vi "_SBR_mes_PM.vi"(6 "SBR_Set":T3={"file_name"="", "HOT/COLD AUTO"=TRUE, "MPI SSB Set"=TRUE, "AUTO時待ち時間（S）"=1.0, "P/V         V/P"=FALSE, "save"=TRUE, "start(GHz)"=4.0, "stop(GHz) "=12.0, "Step(GHz) "=0.1, "P.M.aveg"=10, "PM        SP"=FALSE, "SP_set"={"start(GHz)"=3.5, "stop(GHz) "=12.5, "BW(MHz)"=8.0, "VBW(Hz)"=30.0, "ref(dBm)"=-45.0, "log(dB)"=1.0, "AVEG"=1, "AVEG ON/OFF"=FALSE, "Auto Align ON/OFF"=FALSE, "GPIB"="18", "point"=801}}, 7 "Control":T2={"GPIB_ATT"="28", "6501Dev#"=1, "GPIB_SP"="18", "GPIB_PM"="13", "GPIB_DSA"="11", "GPIB_DMM (TPD)"="23", "MPICOM"="COM5", "mortor設定"=[{"Axis"=0, "ID"=0, "HIspeed"=200.0, "LOspeed"=100.0, "ACCEL(ms)"=100.0, "Sratio"=50.0, "フリーラン\n"=FALSE, "文字列"="DSB HOT/COLD"}, {"Axis"=1, "ID"=0, "HIspeed"=4.0, "LOspeed"=4.0, "ACCEL(ms)"=100.0, "Sratio"=50.0, "フリーラン\n"=TRUE, "文字列"="SubMM Att"}, {"Axis"=0, "ID"=0, "HIspeed"=200.0, "LOspeed"=100.0, "ACCEL(ms)"=100.0, "Sratio"=50.0, "フリーラン\n"=FALSE, "文字列"="MPI Port1"}, {"Axis"=1, "ID"=0, "HIspeed"=200.0, "LOspeed"=100.0, "ACCEL(ms)"=100.0, "Sratio"=50.0, "フリーラン\n"=FALSE, "文字列"="MPI Port2"}], "DATAパス"=path "C:/Documents and Settings/?澤佳?/デスクトップ/data/プロトカ?トリッジ/100811_protC4-5/100814_WCA_P0", "DBパス "=path "Z:/band10/Labview_ALMA/MIX95/test", "comment"="NOLO", "ColdCarts"="003601", "Th"=295.0, "Tc"=77.0, "Set_SIS_volt"=2.096774193548387, "Offset"=0.0, "control"=0, "FreqLO"=796.0, "Set_Mag_Cur"=800.0, "MPI offset(mm)"=22.99, "HOT/COLD"=0} {"HOT/COLD" items=["DSB", "SBR", "GainComp"]; "control" items=["CLOSE LOOP", "OPEN LOOP", "Not Control"]}) -> ()   [LabVIEW 2017]
uses:
  <vilib>/express/express arith-compare/Formula/XNode/ExpressFormulaBlockNode.xnode
panel:
  out "XYグラフ 5":cluster{"データ配列":dbl[], "データ配列":dbl[]}[](graph)
  out "XYグラフ 3":cluster{"データ配列":dbl[], "データ配列":dbl[]}[](graph)=[{"データ配列"=[846.0, 845.9, 845.8, 845.7, 845.6, 845.5, 845.4, 845.3, 845.2, 845.1, 845.0, 844.9, 844.8, 844.7, 844.6, 844.5, 844.4, 844.3, 844.2, 844.1, 844.0, 843.9, 843.8, 843.7, 843.6, 843.5, 843.4, 843.3, 843.2, 843.1, 843.0, 842.9, 842.8, 842.7, 842.6, 842.5, 842.4, 842.3, 842.2, 842.1, 842.0, 841.9, 841.8, 841.7, 841.6, 841.5, 841.4, 841.3, 841.2, 841.1, 841.0, 840.9, 840.8, 840.7, 840.6, 840.5, 840.4, 840.3, 840.2, 840.1, 840.0, 839.9, 839.8, 839.7, 839.6, 839.5, 839.4, 839.3, 839.2, 839.1, 839.0, 838.9, 838.8, 838.7, 838.6, 838.5, 838.4, 838.3, 838.2, 838.1, 838.0], "データ配列"=[548.6440300868269, 532.3446978159301, 548.2566145023541, 544.9061292459833, 538.3138371670094, 526.7499707435629, 519.9997703838006, 527.593359910926, 538.6649629641214, 528.8783476971857, 531.9759636549385, 528.4548463210765, 513.5100557424433, 516.344277513952, 524.5874165109195, 514.3547194297134, 503.7653656940615, 515.5843212692465, 511.0783598537313, 507.55375171659057, 505.8555142030906, 497.52972774878066, 501.23367501224743, 498.1244938121795, 489.8630053526426, 493.1999495623687, 486.236254971209, 488.3096964717638, 482.9518498217425, 485.03073723710247, 486.70267213607735, 480.58951323335924, 482.1108023321396, 481.7962553542322, 480.2342668763604, 480.1246358814105, 478.34749024616036, 479.50312619911205, 480.8342642556151, 480.11632993657906, 480.09010262034064, 481.33419008499317, 479.94632437429556, 479.2444411258671, 475.56007043143904, 479.92516925660385, 474.2701582066877, 475.40266728367556, 479.1159951944159, 479.7010196459051, 475.52458759109373, 472.89567054194913, 473.80662563539966, 472.1704784340717, 468.6585989006322, 468.80409014491283, 479.386903232559, 475.6610934283412, 469.07237974406974, 469.8923820760799, 485.7474282618513, 474.9909858241797, 477.7451890508568, 471.7345659278333, 466.80799840032967, 476.31289425549187, 474.0855612238338, 468.51643935953587, 465.4725917144067, 464.39387004779314, 455.68701805229597, 487.4824379927386, 486.6396397044617, 482.6491011961885, 476.185717770886, 473.69367551401047, 469.2462719814977, 490.9878049262109, 488.417091028331, 483.2977332637604, 478.73867571328907]}, {"データ配列"=[854.0, 854.1, 854.2, 854.3, 854.4, 854.5, 854.6, 854.7, 854.8, 854.9, 855.0, 855.1, 855.2, 855.3, 855.4, 855.5, 855.6, 855.7, 855.8, 855.9, 856.0, 856.1, 856.2, 856.3, 856.4, 856.5, 856.6, 856.7, 856.8, 856.9, 857.0, 857.1, 857.2, 857.3, 857.4, 857.5, 857.6, 857.7, 857.8, 857.9, 858.0, 858.1, 858.2, 858.3, 858.4, 858.5, 858.6, 858.7, 858.8, 858.9, 859.0, 859.1, 859.2, 859.3, 859.4, 859.5, 859.6, 859.7, 859.8, 859.9, 860.0, 860.1, 860.2, 860.3, 860.4, 860.5, 860.6, 860.7, 860.8, 860.9, 861.0, 861.1, 861.2, 861.3, 861.4, 861.5, 861.6, 861.7, 861.8, 861.9, 862.0], "データ配列"=[428.63466788231324, 435.4935786985518, 424.9429241146229, 425.381002919813, 433.20647623071613, 438.7104620965752, 443.67374232684676, 442.41046901070797, 430.10206610123777, 440.4868132571015, 435.759630172149, 438.12370344225775, 449.17411817434277, 446.7229210528855, 440.15843962648995, 446.8897154052984, 455.8583559850793, 448.5867165832221, 448.7198763169121, 459.213527054518, 453.52958129721236, 461.1908621778645, 460.27576536783874, 460.2582724546055, 466.0864670209972, 465.7857212585232, 472.4310313017354, 469.17709649506514, 472.78362850317023, 474.8300149659003, 470.5899912757829, 476.0942267925349, 475.8579793140339, 477.7303156869513, 475.74400495243003, 477.79647352046953, 480.42504158528186, 480.43932637294694, 476.7091000205245, 476.62383716173747, 478.55303619667967, 475.9076566852461, 479.478478145908, 479.03123367121594, 482.39234918165187, 479.54022383471187, 482.5907823874182, 481.7505278760315, 473.16388160930836, 478.15362306779105, 480.4224566467349, 486.5333822347131, 481.63681143700416, 483.9492838089557, 486.8070352464491, 488.59582820525645, 476.5343014109415, 481.9312913888416, 483.0061248872076, 487.93423410039685, 474.129463031071, 479.9925386625467, 481.15577320464706, 486.42199876382404, 486.19935785269905, 480.1111428291795, 482.85166491000814, 488.0712289584561, 488.79712182957707, 494.7195539445724, 498.2972613667672, 469.3853698503216, 471.69756792095194, 474.9496602642304, 474.9261101258189, 481.58901751620425, 485.18240521858206, 464.0725253238966, 468.63537032154585, 470.95286464714934, 473.82427991781964]}]
  out "XYグラフ 2":cluster{"データ配列":dbl[], "データ配列":dbl[]}[](graph)=[{"データ配列"=[4.0, 4.1, 4.2, 4.3, 4.4, 4.5, 4.6, 4.7, 4.8, 4.9, 5.0, 5.1, 5.2, 5.3, 5.4, 5.5, 5.6, 5.7, 5.8, 5.9, 6.0, 6.1, 6.2, 6.3, 6.4, 6.5, 6.6, 6.7, 6.8, 6.9, 7.0, 7.1, 7.2, 7.3, 7.4, 7.5, 7.6, 7.7, 7.8, 7.9, 8.0, 8.1, 8.2, 8.3, 8.4, 8.5, 8.6, 8.7, 8.8, 8.9, 9.0, 9.1, 9.2, 9.3, 9.4, 9.5, 9.6, 9.7, 9.8, 9.9, 10.0, 10.1, 10.2, 10.3, 10.4, 10.5, 10.6, 10.7, 10.8, 10.9, 11.0, 11.1, 11.2, 11.3, 11.4, 11.5, 11.6, 11.7, 11.8, 11.9, 12.0], "データ配列"=[0.9249046199806905, 0.7517460823312963, 0.9540395840198505, 0.9269162846964503, 0.8135071464293695, 0.6845118078872291, 0.5940848741555105, 0.6595267429496003, 0.8424905890766325, 0.6848614491447951, 0.7468632569240828, 0.7017022540247116, 0.5009781568393058, 0.5420517670471693, 0.6567512705093524, 0.5260819433781404, 0.3738892851233047, 0.5210577608576411, 0.4868080144723247, 0.3748668646829679, 0.40851305214688144, 0.2837618549546105, 0.31906128888492447, 0.29578752754072546, 0.186091340659989, 0.21398760146405285, 0.10777417863579805, 0.149529503683046, 0.07958880444948759, 0.07954748815261764, 0.1259459192415544, 0.03515471930494699, 0.048843010718681204, 0.03171586659857754, 0.03513774392157607, 0.01818671370440185, -0.01621661399776954, -0.007299958166486085, 0.03223525679436591, 0.02731107388958061, 0.01199917327442536, 0.042416189630546657, 0.003649695010670608, 0.0016649617408312201, -0.05337023868420484, 0.003002871580193121, -0.06506068611910158, -0.049621795287776015, 0.046733111271247955, 0.012088382838128539, -0.038328518852154166, -0.10639347213811458, -0.061303944619701796, -0.09216414898512537, -0.14209487210153343, -0.15469411614691805, 0.022323601941448917, -0.04899532047290484, -0.10942566444854036, -0.14096019154058603, 0.0905989021163112, -0.0391739187880516, -0.026618766005445365, -0.11471481804298753, -0.1521656000206294, -0.02971053894241202, -0.06853941673839113, -0.15295352656935207, -0.18282933440970475, -0.23669712055460096, -0.33420193764281625, 0.14151372779511212, 0.11668493408571631, 0.06016340251879209, 0.00990019059975937, -0.06182303914612333, -0.12488763229092192, 0.2108352941071432, 0.1546641658899227, 0.09675663767559298, 0.0385754646352136]}, {"データ配列"=[4.0, 4.1, 4.2, 4.3, 4.4, 4.5, 4.6, 4.7, 4.8, 4.9, 5.0, 5.1, 5.2, 5.3, 5.4, 5.5, 5.6, 5.7, 5.8, 5.9, 6.0, 6.1, 6.2, 6.3, 6.4, 6.5, 6.6, 6.7, 6.8, 6.9, 7.0, 7.1, 7.2, 7.3, 7.4, 7.5, 7.6, 7.7, 7.8, 7.9, 8.0, 8.1, 8.2, 8.3, 8.4, 8.5, 8.6, 8.7, 8.8, 8.9, 9.0, 9.1, 9.2, 9.3, 9.4, 9.5, 9.6, 9.7, 9.8, 9.9, 10.0, 10.1, 10.2, 10.3, 10.4, 10.5, 10.6, 10.7, 10.8, 10.9, 11.0, 11.1, 11.2, 11.3, 11.4, 11.5, 11.6, 11.7, 11.8, 11.9, 12.0], "データ配列"=[0.8608442548458806, 0.7044947061255087, 0.942586230446133, 0.8493423462533632, 0.7498852904990045, 0.6081560581526015, 0.5430236262647461, 0.6112878364871215, 0.7766440219127979, 0.6149782219119803, 0.6572667110064123, 0.6314153665922547, 0.42698388986216995, 0.42556280195907853, 0.6250719853321322, 0.46430207183002675, 0.33449694284816134, 0.3882474607513784, 0.41506556549956136, 0.3095955000245737, 0.3439051059443347, 0.18240325622893133, 0.28216500097201935, 0.21140353248088684, 0.09413496569057882, 0.17821059451244267, 0.02989001559470223, 0.08828842570711844, 0.050866182648811285, 0.05573387700815249, 0.0663662835217892, 0.0060675597842494156, 0.025335116139840193, -0.04466065840811484, -0.0009333943257959284, -0.05014719752768275, -0.03863850457661142, -0.05952305731929579, -0.037721361400900405, -0.057166062404831075, -0.02916814808995304, -0.012193201434749976, -0.05312032998266237, -0.03611908754398227, -0.1487916724233145, -0.0936345982389959, -0.11305505580370279, -0.1339112513602761, -0.06524335069777229, -0.05628499636478335, -0.11671426437024365, -0.12007755334931655, -0.07430213142730542, -0.1433316372459072, -0.19742493600277894, -0.24364724201221805, -0.08095792610453033, -0.11881261902412663, -0.18295836886949077, -0.1796637370590902, -0.0021771227974171498, -0.026775088377075353, -0.0733922953710137, -0.21148011251519863, -0.21732805814513603, -0.10245993628641197, -0.15420496911591877, -0.19693792604968408, -0.25066612288482537, -0.32217008482607234, -0.39040508822987946, 0.10341354358296367, 0.0815119128548301, -0.0023439054432579094, -0.09006479558012595, -0.1407232856746613, -0.1823207569229413, 0.17679562449456773, 0.08239435268162094, 0.017011997383429706, -0.016509469169492315]}]
  out "XYグラフ 4":cluster{"データ配列":dbl[], "データ配列":dbl[]}[](graph)=[{"データ配列"=[4.0, 4.1, 4.2, 4.3, 4.4, 4.5, 4.6, 4.7, 4.8, 4.9, 5.0, 5.1, 5.2, 5.3, 5.4, 5.5, 5.6, 5.7, 5.8, 5.9, 6.0, 6.1, 6.2, 6.300000000000001, 6.4, 6.5, 6.6, 6.7, 6.800000000000001, 6.9, 7.0, 7.1, 7.2, 7.300000000000001, 7.4, 7.5, 7.6, 7.7, 7.800000000000001, 7.9, 8.0, 8.100000000000001, 8.2, 8.3, 8.4, 8.5, 8.600000000000001, 8.7, 8.8, 8.9, 9.0, 9.100000000000001, 9.2, 9.3, 9.4, 9.5, 9.600000000000001, 9.7, 9.8, 9.9, 10.0, 10.100000000000001, 10.2, 10.3, 10.4, 10.5, 10.600000000000001, 10.7, 10.8, 10.9, 11.0, 11.100000000000001, 11.2, 11.3, 11.4, 11.5, 11.600000000000001, 11.7, 11.8, 11.9, 12.0], "データ配列"=[-12.8167177, -12.8141441, -12.8129357, -12.8127695, -12.8146098, -12.8149315, -12.8129768, -12.8171079, -12.8151768, -12.8168376, -12.8133399, -12.8138484, -12.8165291, -12.82274, -12.8215599, -12.8278529, -12.8327051, -12.84042, -12.8387483, -12.8518869, -12.8490208, -12.8535159, -12.8552697, -12.8598767, -12.8577317, -12.8589288, -12.8659834, -12.8643617, -12.866542, -12.8707753, -12.8715886, -12.8749385, -12.8803226, -12.8889543, -12.888898, -12.8977837, -12.8968323, -12.9040674, -12.9085005, -12.9114525, -12.9163973, -12.910995, -12.9094349, -12.9092876, -12.9091013, -12.9068352, -12.9020569, -12.9040377, -12.8989597, -12.899771, -12.8980538, -12.8942882, -12.8828067, -12.8807576, -12.8755902, -12.8728258, -12.8664256, -12.8622031, -12.85197, -12.8488996, -12.8492387, -12.838981799999999, -12.8414434, -12.8447165, -12.8376775, -12.840512, -12.8396292, -12.8369379, -12.8346457, -12.8405822, -12.8328279, -12.8329255, -12.8308305, -12.8282862, -12.8235474, -12.821384, -12.8175541, -12.8162696, -12.8153706, -12.8112541, -12.8080699]}, {"データ配列"=[4.0, 4.1, 4.2, 4.3, 4.4, 4.5, 4.6, 4.7, 4.8, 4.9, 5.0, 5.1, 5.2, 5.3, 5.4, 5.5, 5.6, 5.7, 5.8, 5.9, 6.0, 6.1, 6.2, 6.300000000000001, 6.4, 6.5, 6.6, 6.7, 6.800000000000001, 6.9, 7.0, 7.1, 7.2, 7.300000000000001, 7.4, 7.5, 7.6, 7.7, 7.800000000000001, 7.9, 8.0, 8.100000000000001, 8.2, 8.3, 8.4, 8.5, 8.600000000000001, 8.7, 8.8, 8.9, 9.0, 9.100000000000001, 9.2, 9.3, 9.4, 9.5, 9.600000000000001, 9.7, 9.8, 9.9, 10.0, 10.100000000000001, 10.2, 10.3, 10.4, 10.5, 10.600000000000001, 10.7, 10.8, 10.9, 11.0, 11.100000000000001, 11.2, 11.3, 11.4, 11.5, 11.600000000000001, 11.7, 11.8, 11.9, 12.0], "データ配列"=[-13.7683758, -13.7922764, -13.7633268, -13.7678909, -13.7828507, -13.8025731, -13.8131615, -13.8053932, -13.7812508, -13.8023359, -13.7920552, -13.7989576, -13.8295585, -13.8300327, -13.8131129, -13.8384301, -13.8642177, -13.8495674, -13.8552811, -13.8790433, -13.8758927, -13.8977266, -13.892538, -13.9026757, -13.916412, -13.9124923, -13.9338423, -13.9277004, -13.9399338, -13.9424098, -13.9378287, -13.9546529, -13.9572289, -13.9670513, -13.969147, -13.9785946, -13.9824585, -13.9877933, -13.9872335, -13.9922533, -13.9981255, -13.9884289, -13.9918875, -13.992756, -13.9997441, -13.98919, -13.9960103, -13.9950765, -13.9790547, -13.9820422, -13.9886454, -13.9916958, -13.9764347, -13.9790154, -13.9814203, -13.9784988, -13.9476282, -13.9532534, -13.9552977, -13.9526629, -13.9176991, -13.9298424, -13.9285866, -13.9449108, -13.9459258, -13.927964, -13.9333817, -13.9436702, -13.9472559, -13.9575221, -13.9665371, -13.8965286, -13.8978142, -13.9040012, -13.9102852, -13.9152088, -13.9199899, -13.8711522, -13.8776705, -13.8837972, -13.8899317]}, {"データ配列"=[4.0, 4.1, 4.2, 4.3, 4.4, 4.5, 4.6, 4.7, 4.8, 4.9, 5.0, 5.1, 5.2, 5.3, 5.4, 5.5, 5.6, 5.7, 5.8, 5.9, 6.0, 6.1, 6.2, 6.300000000000001, 6.4, 6.5, 6.6, 6.7, 6.800000000000001, 6.9, 7.0, 7.1, 7.2, 7.300000000000001, 7.4, 7.5, 7.6, 7.7, 7.800000000000001, 7.9, 8.0, 8.100000000000001, 8.2, 8.3, 8.4, 8.5, 8.600000000000001, 8.7, 8.8, 8.9, 9.0, 9.100000000000001, 9.2, 9.3, 9.4, 9.5, 9.600000000000001, 9.7, 9.8, 9.9, 10.0, 10.100000000000001, 10.2, 10.3, 10.4, 10.5, 10.600000000000001, 10.7, 10.8, 10.9, 11.0, 11.100000000000001, 11.2, 11.3, 11.4, 11.5, 11.600000000000001, 11.7, 11.8, 11.9, 12.0], "データ配列"=[-15.3373199, -15.3434384, -15.3418441, -15.3453406, -15.3400846, -15.3458539, -15.3440331, -15.3394241, -15.3465619, -15.3410986, -15.3426298, -15.3434557, -15.346694, -15.3533297, -15.3527599, -15.3611371, -15.3653082, -15.3685527, -15.3735164, -15.3722621, -15.3827205, -15.3861695, -15.3836614, -15.3932886, -15.3939993, -15.3902446, -15.3969746, -15.3976586, -15.402461, -15.3995764, -15.4050633, -15.4090926, -15.4122846, -15.4181912, -15.4242723, -15.4297683, -15.4273514, -15.4325704, -15.4411621, -15.4454937, -15.4471412, -15.4441903, -15.4388196, -15.4406587, -15.4410973, -15.4361552, -15.4359821, -15.4374129, -15.4407749, -15.4318682, -15.4334771, -15.4239621, -15.4191743, -15.4160723, -15.4123312, -15.4063207, -15.4018825, -15.3948126, -15.3943757, -15.3815451, -15.378063, -15.3760794, -15.371747, -15.3766317, -15.3787598, -15.3750977, -15.3734286, -15.3718175, -15.3738011, -15.3719326, -15.3744687, -15.3672418, -15.3624387, -15.360924, -15.3673373, -15.3580207, -15.3559741, -15.3543332, -15.3494625, -15.3498174, -15.3493734]}, {"データ配列"=[4.0, 4.1, 4.2, 4.3, 4.4, 4.5, 4.6, 4.7, 4.8, 4.9, 5.0, 5.1, 5.2, 5.3, 5.4, 5.5, 5.6, 5.7, 5.8, 5.9, 6.0, 6.1, 6.2, 6.300000000000001, 6.4, 6.5, 6.6, 6.7, 6.800000000000001, 6.9, 7.0, 7.1, 7.2, 7.300000000000001, 7.4, 7.5, 7.6, 7.7, 7.800000000000001, 7.9, 8.0, 8.100000000000001, 8.2, 8.3, 8.4, 8.5, 8.600000000000001, 8.7, 8.8, 8.9, 9.0, 9.100000000000001, 9.2, 9.3, 9.4, 9.5, 9.600000000000001, 9.7, 9.8, 9.9, 10.0, 10.100000000000001, 10.2, 10.3, 10.4, 10.5, 10.600000000000001, 10.7, 10.8, 10.9, 11.0, 11.100000000000001, 11.2, 11.3, 11.4, 11.5, 11.600000000000001, 11.7, 11.8, 11.9, 12.0], "データ配列"=[-14.0196387, -13.9979183, -14.0309121, -14.018873, -14.0036354, -13.9857556, -13.9744838, -13.9850344, -14.0105081, -13.9859785, -13.9904136, -13.9872409, -13.9607929, -13.9671506, -13.9949353, -13.9786552, -13.9646952, -13.9787962, -13.9830638, -13.9758055, -13.9829474, -13.9637367, -13.9786938, -13.9745032, -13.9572288, -13.9680508, -13.9544577, -13.9613969, -13.9599726, -13.9615707, -13.9660668, -13.960714, -13.9681177, -13.9661289, -13.9740149, -13.975349, -13.9750328, -13.9785234, -13.9884027, -13.9882046, -13.9960013, -13.9947386, -13.9851271, -13.9880813, -13.9730589, -13.9769712, -13.9707784, -13.9701434, -13.9780513, -13.9759535, -13.96688, -13.9613857, -13.9585451, -13.9457407, -13.9334979, -13.9238702, -13.9411322, -13.9297898, -13.9138048, -13.9083049, -13.933475, -13.9215995, -13.9145318, -13.8989468, -13.8948861, -13.9126915, -13.9031456, -13.8942396, -13.8858065, -13.8794991, -13.8666928, -13.9337306, -13.926695, -13.9122424, -13.8990967, -13.8877931, -13.8797191, -13.9291645, -13.9124584, -13.900162, -13.8931044]}, {"データ配列"=[4.0, 4.1, 4.2, 4.3, 4.4, 4.5, 4.6, 4.7, 4.8, 4.9, 5.0, 5.1, 5.2, 5.3, 5.4, 5.5, 5.6, 5.7, 5.8, 5.9, 6.0, 6.1, 6.2, 6.300000000000001, 6.4, 6.5, 6.6, 6.7, 6.800000000000001, 6.9, 7.0, 7.1, 7.2, 7.300000000000001, 7.4, 7.5, 7.6, 7.7, 7.800000000000001, 7.9, 8.0, 8.100000000000001, 8.2, 8.3, 8.4, 8.5, 8.600000000000001, 8.7, 8.8, 8.9, 9.0, 9.100000000000001, 9.2, 9.3, 9.4, 9.5, 9.600000000000001, 9.7, 9.8, 9.9, 10.0, 10.100000000000001, 10.2, 10.3, 10.4, 10.5, 10.600000000000001, 10.7, 10.8, 10.9, 11.0, 11.100000000000001, 11.2, 11.3, 11.4, 11.5, 11.600000000000001, 11.7, 11.8, 11.9, 12.0], "データ配列"=[-15.3381941, -15.344199, -15.3447699, -15.3425074, -15.3371397, -15.3411604, -15.3414315, -15.3458022, -15.3417021, -15.3392578, -15.3397076, -15.3444271, -15.3474302, -15.3513504, -15.3547842, -15.3633021, -15.3614004, -15.3666426, -15.3702935, -15.3730672, -15.379985, -15.3834281, -15.3866312, -15.3912841, -15.3891415, -15.3940469, -15.3981261, -15.3947827, -15.3998376, -15.4000821, -15.408751, -15.4094613, -15.4119679, -15.417087, -15.4276622, -15.4229367, -15.429126, -15.4411081, -15.4378729, -15.4476114, -15.4489349, -15.4440339, -15.44137, -15.4421306, -15.434502, -15.4333984, -15.4405416, -15.4352283, -15.4339626, -15.4288343, -15.4309286, -15.422514, -15.4216582, -15.4149915, -15.4117796, -15.3984203, -15.4001348, -15.3945141, -15.3895448, -15.3827213, -15.3762016, -15.3734612, -15.3759497, -15.3702058, -15.3743928, -15.3765457, -15.3732681, -15.3712204, -15.3747897, -15.3710142, -15.3719226, -15.3681146, -15.3646886, -15.3646273, -15.3572943, -15.3592383, -15.3537235, -15.354729, -15.3478549, -15.3463945, -15.3471664]}]
  out "文字列":string="19.85991\r\n"
  in  "Tin":T1(ring)
  in  "OKボタン":bool=TRUE
  in  "タブ制御器":enum32{"ページ 5", "ページ 2", "ページ 4"}(tab)
  out "MPI SBR(dB)":dbl=19.65107286127357
  out "MU（mag）":dbl=0.6324558993924078
  out "ML（mag）":dbl=0.006853666405205144
  out "MPIPOS（mm）":dbl=19.85991633178654
  out "1Dデータ":dbl[](array[numeric])=[12.0, -12.8080699, -13.8899317, -15.3493734, -13.8931044, -15.3471664, 19.85991633178654, 0.0]
  out "SBRAクラスタ":T4={"データ配列"=array801x17[13617 elements], "Points"=801, "Th"=297.0, "Tc"=77.0, "LO(GHz)"=0.0, "Offset(mm)"=0.0, "Pos(mm)"=0.0, "P/V         V/P"=FALSE, "AUTOSAVE"=TRUE, "file_name"="", "パス"=path "", "header+(filename)"="A_"}
  # "Port"
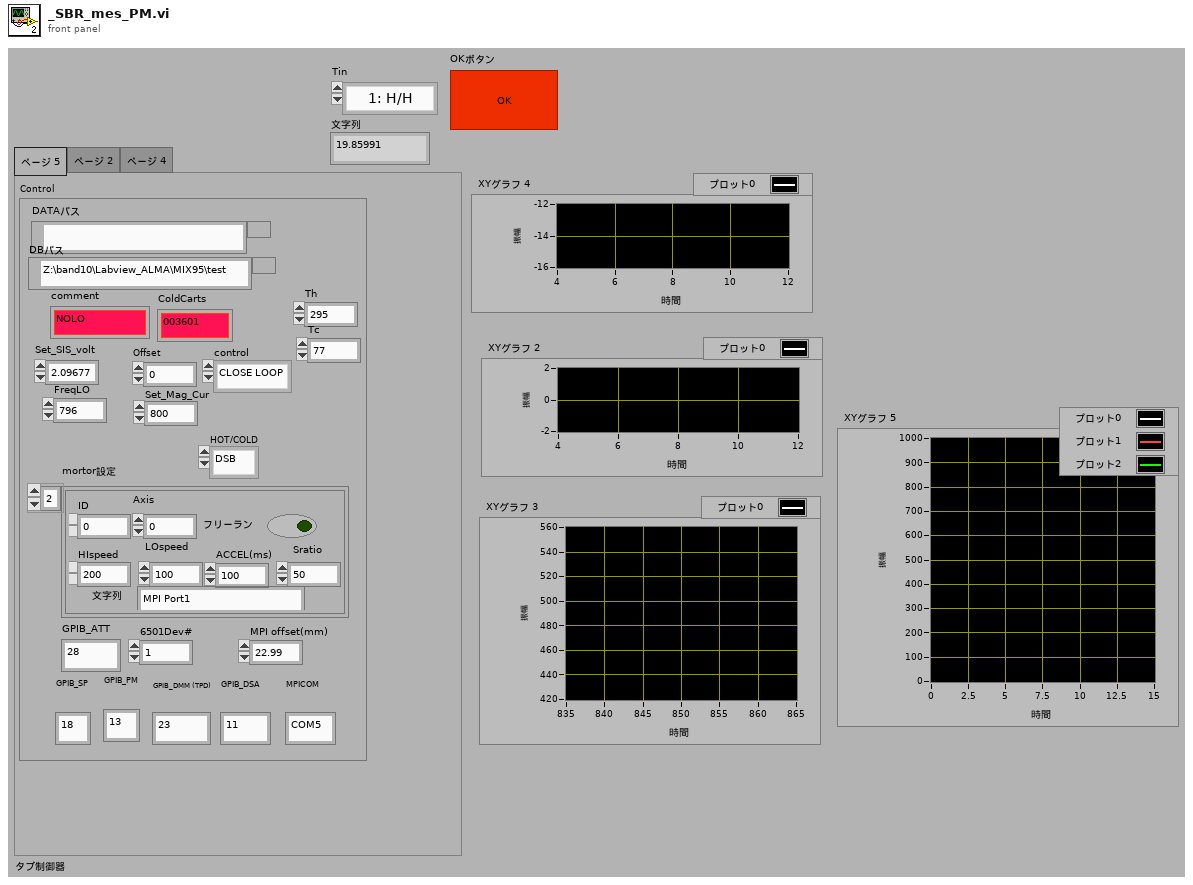
[diagram p1: front panel]
types:
  T1 = enum16{"1: H/H", "2: H/C", "3: C/C", "4: C/H", "5: H/H"}
  T2 = cluster{"GPIB_ATT":string, "6501Dev#":i16, "GPIB_SP":string, "GPIB_PM":string, "GPIB_DSA":string, "GPIB_DMM (TPD)":string, "MPICOM":string, "mortor設定":cluster{"Axis":i16, "ID":i16, "HIspeed":dbl, "LOspeed":dbl, "ACCEL(ms)":dbl, "Sratio":dbl, "フリーラン\n":bool, "文字列":string}[], "DATAパス":path, "DBパス ":path, "comment":string, "ColdCarts":string, "Th":dbl, "Tc":dbl, "Set_SIS_volt":dbl, "Offset":dbl, "control":u16, "FreqLO":dbl, "Set_Mag_Cur":dbl, "MPI offset(mm)":dbl, "HOT/COLD":u16}
  T3 = cluster{"file_name":string, "HOT/COLD AUTO":bool, "MPI SSB Set":bool, "AUTO時待ち時間（S）":dbl, "P/V         V/P":bool, "save":bool, "start(GHz)":dbl, "stop(GHz) ":dbl, "Step(GHz) ":dbl, "P.M.aveg":i32, "PM        SP":bool, "SP_set":cluster{"start(GHz)":dbl, "stop(GHz) ":dbl, "BW(MHz)":dbl, "VBW(Hz)":dbl, "ref(dBm)":dbl, "log(dB)":dbl, "AVEG":i16, "AVEG ON/OFF":bool, "Auto Align ON/OFF":bool, "GPIB":string, "point":i16}}
  T4 = cluster{"データ配列":dbl[][], "Points":i32, "Th":dbl, "Tc":dbl, "LO(GHz)":dbl, "Offset(mm)":dbl, "Pos(mm)":dbl, "P/V         V/P":bool, "AUTOSAVE":bool, "file_name":string, "パス":path, "header+(filename)":string}
  T5 = cluster{"Axis":i16, "ID":i16, "HIspeed":dbl, "LOspeed":dbl, "ACCEL(ms)":dbl, "Sratio":dbl, "フリーラン\n":bool, "文字列":string}[]
  T6 = cluster{"Axis":i16, "ID":i16, "HIspeed":dbl, "LOspeed":dbl, "ACCEL(ms)":dbl, "Sratio":dbl, "フリーラン\n":bool, "文字列":string}
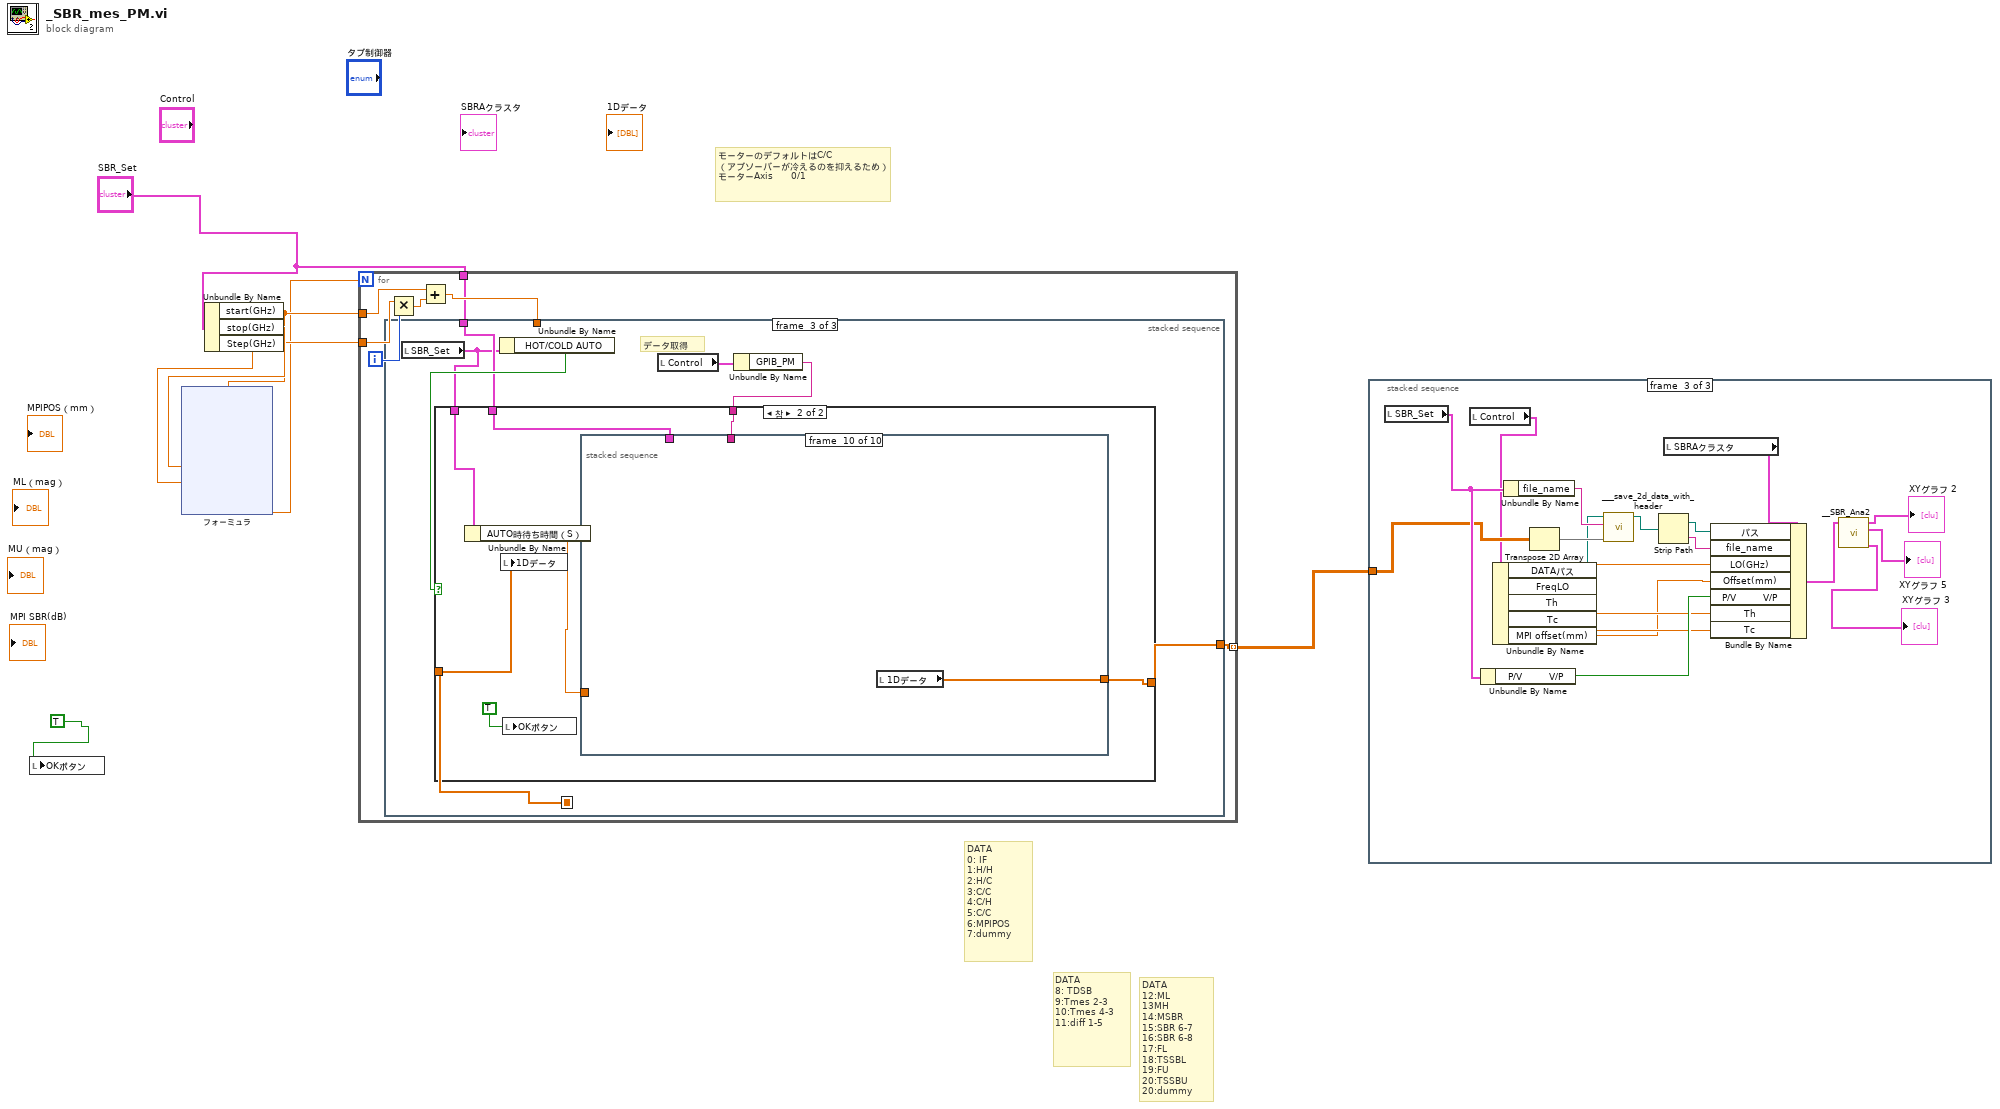
[diagram p0: block diagram]
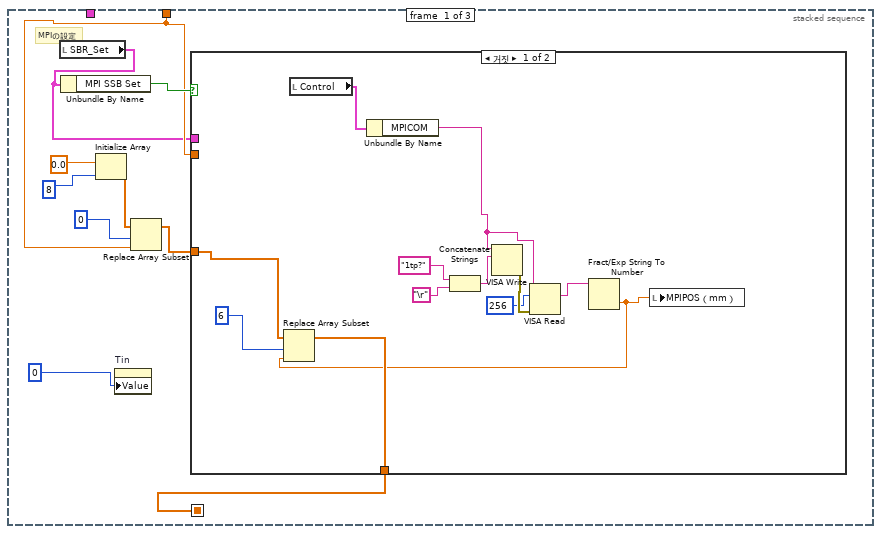
[diagram p2: hidden frame]
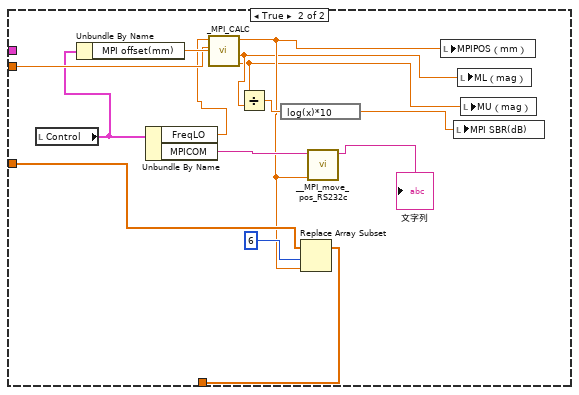
[diagram p3: hidden frame]
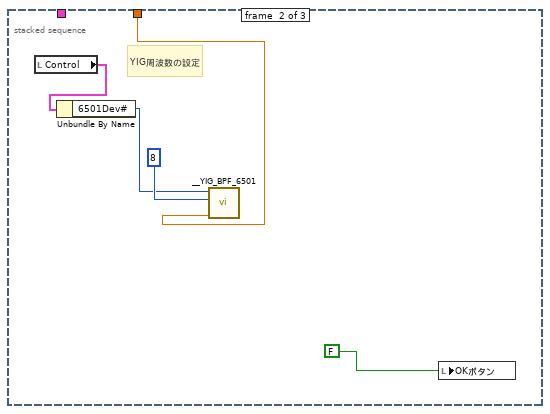
[diagram p4: hidden frame]
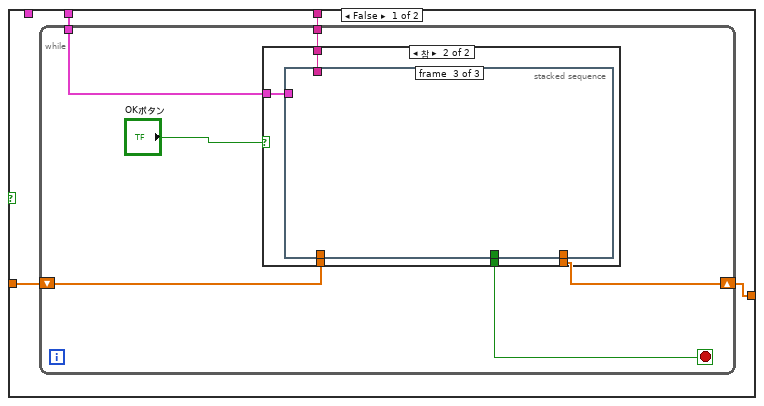
[diagram p5: hidden frame]
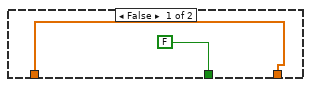
[diagram p6: hidden frame]
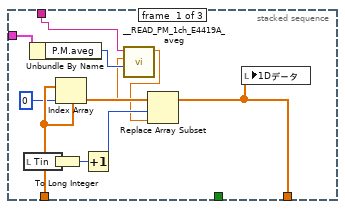
[diagram p7: hidden frame]
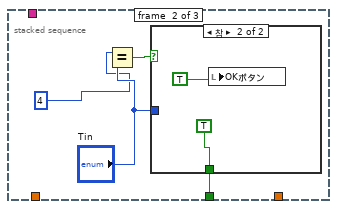
[diagram p8: hidden frame]
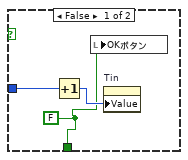
[diagram p9: hidden frame]
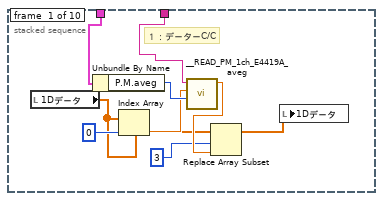
[diagram p10: hidden frame]
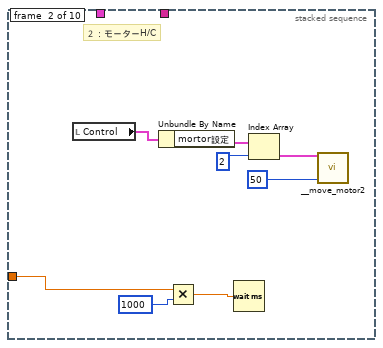
[diagram p11: hidden frame]
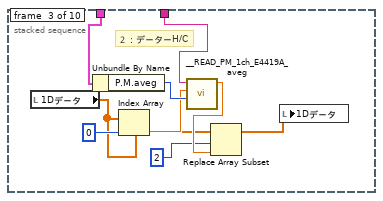
[diagram p12: hidden frame]
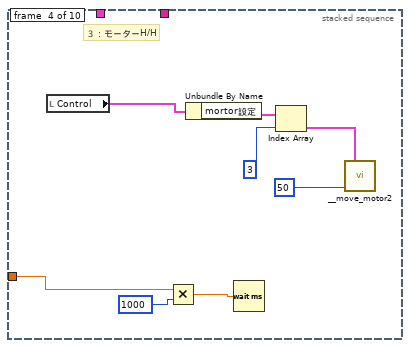
[diagram p13: hidden frame]
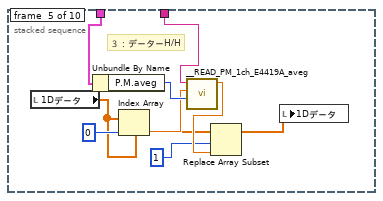
[diagram p14: hidden frame]
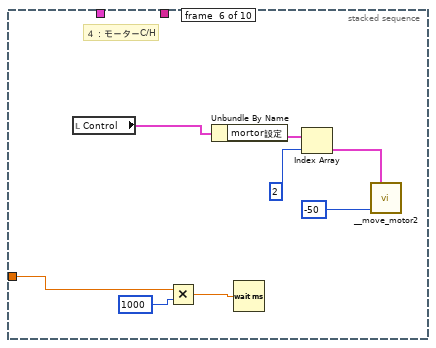
[diagram p15: hidden frame]
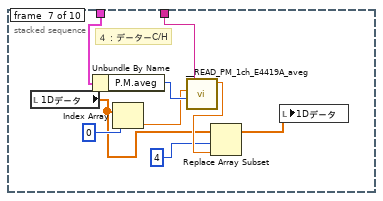
[diagram p16: hidden frame]
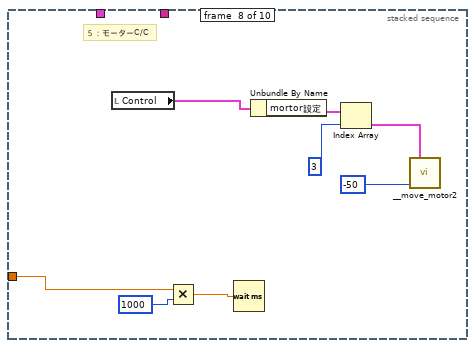
[diagram p17: hidden frame]
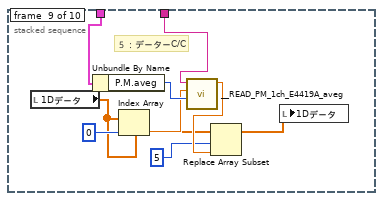
[diagram p18: hidden frame]
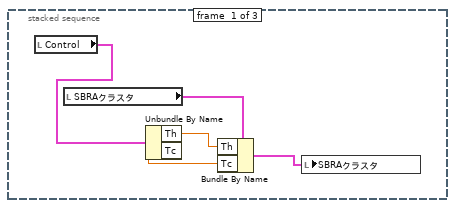
[diagram p19: hidden frame]
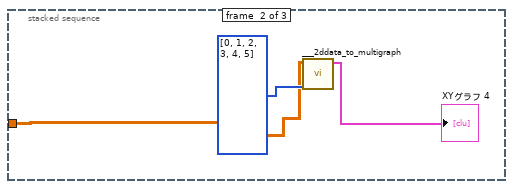
[diagram p20: hidden frame]
diagram:
  # "DATA\n0: IF\n1:H/H\n2:H/C\n3:C/C\n4:C/H\n5:C/C\n6:MPIPOS\n7:dummy"
  # "DATA\n12:ML\n13MH\n14:MSBR\n15:SBR 6-7\n16:SBR 6-8\n17:FL\n18:TSSBL\n19:FU\n20:TSSBU\n20:dummy"
  # "DATA\n8: TDSB\n9:Tmes 2-3\n10:Tmes 4-3\n11:diff 1-5"
  # "モーターのデフォルトはC/C\n（アブソーバーが冷えるのを抑えるため）\nモーターAxis　　0/1"
  n1 = local write "OKボタン"(TRUE) -> ()
  n2 = Unbundle By Name("SBR_Set") -> ("start(GHz)"=w3:dbl, "stop(GHz)"=w4:dbl, "Step(GHz)"=w2:dbl)
  n3 = xnode "フォーミュラ"("start"=w3, "stop"=w4, "step"=w2) -> ("結果"=w1:dbl)  [unwired: 1 in, 1 out]
  n4 = for {
    N: w1 -> [_]
    tunnel: w3 -> [w14]
    tunnel: w2 -> [w12]
    tunnel: "SBR_Set" -> [w9]
    tunnel: [w8] -> w6 mode=indexing
    i -> [w11]
    n5 = Multiply(x=w12, y=w11) -> (x*y=w13:dbl)
    n6 = Add(x=w14, y=w13) -> (x+y=w10:dbl)
    n7 = stacked-sequence {
      seq-local: [w15 _ _] -> [_ _ w62]
      tunnel: w10 -> [w19 w53 _]
      tunnel: w9 -> [_ _ w60]
      tunnel: [_ _ w59] -> w8
      frame #0 {
        # "MPIの設定"
        n8 = local read "SBR_Set"() -> (w17:T3)
        n9 = Unbundle By Name(w17) -> ("MPI SSB Set"=w24:bool)
        n10 = Initialize Array(0.0, 8) -> (w21:dbl[])
        n11 = property on="Tin" class="Enum (决拜茄)"("Value"=0) -> ()  [unwired: 2 in, 2 out]
        n12 = Replace Array Subset(array=w21, new element=w19, index=0) -> (w16:dbl[])
        n13 = case shown="거짓" w24 {
          tunnel: w17 -> [_ _]
          tunnel: w19 -> [_ w48]
          tunnel: w16 -> [w32 w45]
          tunnel: [w33 w44] -> w15
          frame False {
            n14 = local read "Control"() -> (w29:T2)
            n15 = Unbundle By Name(w29) -> ("MPICOM"=w36:string)
            n16 = Concatenate Strings("1tp?", "\r") -> (w26:string)
            n17 = VISA Write(VISA resource name=w36, write buffer=w26) -> (error out=w35:errorcluster)  [unwired: 1 in, 2 out]
            n18 = VISA Read(VISA resource name=w36, byte count=256, error in (no error)=w35) -> (read buffer=w28:string)  [unwired: 3 out]
            n19 = Fract/Exp String To Number(string=w28) -> (number=w30:dbl)  [unwired: 3 in, 1 out]
            n20 = Replace Array Subset(array=w32, new element=w30, index=6) -> (w33:dbl[])
            n21 = local write "MPIPOS（mm）"(w30) -> ()
          }
          frame True {
            n22 = local read "Control"() -> (w37:T2)
            n23 = Unbundle By Name(w37) -> ("MPI offset(mm)"=w50:dbl)
            n24 = Unbundle By Name(w37) -> ("FreqLO"=w42:dbl, "MPICOM"=w43:string)
            n25 = call "_MPI_CALC.vi"("ofset (mm)"=w50, "IF（GHｚ）"=w48, "LO（GHｚ）"=w42) -> ("PU (mag)"=w39:dbl, "PL (lmag)"=w40:dbl, "SSB_pos(mm)"=w41:dbl)  [unwired: 6 in]
            n26 = Divide(x=w39, y=w40) -> (x/y=w49:dbl)
            n27 = expression code="log(x)*10"(w49) -> (w38:dbl)
            n28 = Replace Array Subset(array=w45, new element=w41, index=6) -> (w44:dbl[])
            n29 = call "__MPI_move_pos_RS232c.vi"("pos"=w41, "VISAリソース名"=w43) -> ("動作中現在位置"=→"文字列":string)  [unwired: 5 in]
            n30 = local write "MPIPOS（mm）"(w41) -> ()
            n31 = local write "MPI SBR(dB)"(w38) -> ()
            n32 = local write "ML（mag）"(w40) -> ()
            n33 = local write "MU（mag）"(w39) -> ()
          }
        }
      }
      frame #1 {
        # "YIG周波数の設定"
        n34 = local read "Control"() -> (w51:T2)
        n35 = Unbundle By Name(w51) -> ("6501Dev#"=w54:i16)
        n36 = call "__YIG_BPF_6501.vi"("fc(GHz)"=w53, "bit"=8, "Dev(1,2..)"=w54) -> ()  [unwired: 1 in]
        n37 = local write "OKボタン"(FALSE) -> ()
      }
      frame #2 {
        # "データ取得"
        n38 = local read "SBR_Set"() -> (w58:T3)
        n39 = Unbundle By Name(w58) -> ("HOT/COLD AUTO"=w61:bool)
        n40 = local read "Control"() -> (w57:T2)
        n41 = Unbundle By Name(w57) -> ("GPIB_PM"=w56:string)
        n42 = case shown="참" w61 {
          tunnel: w62 -> [w66 w105]
          tunnel: [w65 w102] -> w59
          tunnel: w60 -> [w64 w106]
          tunnel: w58 -> [_ w104]
          tunnel: w56 -> [w63 w100]
          frame False {
            n43 = while {
              shift-right: [w69] -> w65
              shift-left: w66 -> [w70]
              tunnel: w64 -> [w68]
              tunnel: w63 -> [w67]
              stop <- w72 stop-if-true
              n44 = case shown="참" "OKボタン" {
                tunnel: [FALSE w79] -> w72
                tunnel: w70 -> [w73 w78]
                tunnel: [w73 w76] -> w69
                tunnel: w68 -> [_ w77]
                tunnel: w67 -> [_ w75]
                frame False {
                }
                frame True {
                  n45 = stacked-sequence {
                    tunnel: [_ w93 _] -> w79
                    tunnel: w78 -> [w85 _ _]
                    tunnel: w77 -> [w87 _ _]
                    tunnel: [w81 _ _] -> w76
                    tunnel: w75 -> [w80 _ _]
                    frame #0 {
                      n46 = local read "Tin"() -> (w90:T1)
                      n47 = Unbundle By Name(w87) -> ("P.M.aveg"=w86:i32)
                      n48 = To Long Integer(number=w90) -> (32bit integer=w88:i32)
                      n49 = Index Array(array=w85, index=0) -> (element=w83:dbl)
                      n50 = Increment(x=w88) -> (x+1=w89:i32)
                      n51 = call "__READ_PM_1ch_E4419A_aveg.VI"("aveg"=w86, "frq(GHz)"=w83, "GPIB"=w80) -> ("chA"=w82:dbl)  [unwired: 4 in]
                      n52 = Replace Array Subset(array=w85, new element=w82, index=w89) -> (w81:dbl[])
                      n53 = local write "1Dデータ"(w81) -> ()
                    }
                    frame #1 {
                      n54 = Equal?(x=4, y="Tin") -> (x = y?=w94:bool)
                      n55 = case shown="참" w94 {
                        tunnel: [w95 TRUE] -> w93
                        tunnel: "Tin" -> [w97 _]
                        frame False {
                          w95 = FALSE
                          n56 = Increment(x=w97) -> (x+1=w96:T1)
                          n57 = local write "OKボタン"(w95) -> ()
                          n58 = property on="Tin" class="Enum (决拜茄)"("Value"=w96) -> ()  [unwired: 2 in, 2 out]
                        }
                        frame True {
                          n59 = local write "OKボタン"(TRUE) -> ()
                        }
                      }
                    }
                    frame #2 {
                    }
                  }
                }
              }
            }
          }
          frame True {
            n60 = Unbundle By Name(w104) -> ("AUTO時待ち時間（S）"=w103:dbl)
            n61 = local write "1Dデータ"(w105) -> ()
            n62 = local write "OKボタン"(TRUE) -> ()
            n63 = stacked-sequence {
              tunnel: w106 -> [w111 _ w128 _ w145 _ w162 _ w179 _]
              tunnel: w103 -> [_ w121 _ w138 _ w155 _ w172 _ _]
              tunnel: [_ _ _ _ _ _ _ _ _ w184] -> w102
              tunnel: w100 -> [w107 _ w124 _ w141 _ w158 _ w175 _]
              frame #0 {
                # "１：データーC/C"
                n64 = local read "1Dデータ"() -> (w109:dbl[])
                n65 = Unbundle By Name(w111) -> ("P.M.aveg"=w115:i32)
                n66 = Index Array(array=w109, index=0) -> (element=w113:dbl)
                n67 = call "__READ_PM_1ch_E4419A_aveg.VI"("aveg"=w115, "frq(GHz)"=w113, "GPIB"=w107) -> ("chA"=w112:dbl)  [unwired: 4 in]
                n68 = Replace Array Subset(array=w109, new element=w112, index=3) -> (w108:dbl[])
                n69 = local write "1Dデータ"(w108) -> ()
              }
              frame #1 {
                # "２：モーターH/C"
                n70 = local read "Control"() -> (w120:T2)
                n71 = Unbundle By Name(w120) -> ("mortor設定"=w116:T5)
                n72 = Multiply(x=w121, y=1000) -> (x*y=w123:dbl)
                n73 = Wait (ms)(milliseconds to wait=w123) -> ()  [unwired: 1 out]
                n74 = Index Array(array=w116, index=2) -> (element=w119:T6)
                n75 = call "__move_motor2.vi"("Moving distance"=50, "motor setup"=w119) -> ()  [unwired: 2 in, 2 out]
              }
              frame #2 {
                # "２：データーH/C"
                n76 = local read "1Dデータ"() -> (w126:dbl[])
                n77 = Unbundle By Name(w128) -> ("P.M.aveg"=w132:i32)
                n78 = Index Array(array=w126, index=0) -> (element=w130:dbl)
                n79 = call "__READ_PM_1ch_E4419A_aveg.VI"("aveg"=w132, "frq(GHz)"=w130, "GPIB"=w124) -> ("chA"=w129:dbl)  [unwired: 4 in]
                n80 = Replace Array Subset(array=w126, new element=w129, index=2) -> (w125:dbl[])
                n81 = local write "1Dデータ"(w125) -> ()
              }
              frame #3 {
                # "３：モーターH/H"
                n82 = local read "Control"() -> (w137:T2)
                n83 = Multiply(x=w138, y=1000) -> (x*y=w140:dbl)
                n84 = Unbundle By Name(w137) -> ("mortor設定"=w133:T5)
                n85 = Wait (ms)(milliseconds to wait=w140) -> ()  [unwired: 1 out]
                n86 = Index Array(array=w133, index=3) -> (element=w136:T6)
                n87 = call "__move_motor2.vi"("Moving distance"=50, "motor setup"=w136) -> ()  [unwired: 2 in, 2 out]
              }
              frame #4 {
                # "３：データーH/H"
                n88 = local read "1Dデータ"() -> (w143:dbl[])
                n89 = Unbundle By Name(w145) -> ("P.M.aveg"=w149:i32)
                n90 = Index Array(array=w143, index=0) -> (element=w147:dbl)
                n91 = call "__READ_PM_1ch_E4419A_aveg.VI"("aveg"=w149, "frq(GHz)"=w147, "GPIB"=w141) -> ("chA"=w146:dbl)  [unwired: 4 in]
                n92 = Replace Array Subset(array=w143, new element=w146, index=1) -> (w142:dbl[])
                n93 = local write "1Dデータ"(w142) -> ()
              }
              frame #5 {
                # "４：モーターC/H"
                n94 = local read "Control"() -> (w154:T2)
                n95 = Multiply(x=w155, y=1000) -> (x*y=w157:dbl)
                n96 = Unbundle By Name(w154) -> ("mortor設定"=w150:T5)
                n97 = Wait (ms)(milliseconds to wait=w157) -> ()  [unwired: 1 out]
                n98 = Index Array(array=w150, index=2) -> (element=w153:T6)
                n99 = call "__move_motor2.vi"("Moving distance"=-50, "motor setup"=w153) -> ()  [unwired: 2 in, 2 out]
              }
              frame #6 {
                # "４：データーC/H"
                n100 = local read "1Dデータ"() -> (w160:dbl[])
                n101 = Unbundle By Name(w162) -> ("P.M.aveg"=w166:i32)
                n102 = Index Array(array=w160, index=0) -> (element=w164:dbl)
                n103 = call "__READ_PM_1ch_E4419A_aveg.VI"("aveg"=w166, "frq(GHz)"=w164, "GPIB"=w158) -> ("chA"=w163:dbl)  [unwired: 4 in]
                n104 = Replace Array Subset(array=w160, new element=w163, index=4) -> (w159:dbl[])
                n105 = local write "1Dデータ"(w159) -> ()
              }
              frame #7 {
                # "５：モーターC/C"
                n106 = local read "Control"() -> (w171:T2)
                n107 = Multiply(x=w172, y=1000) -> (x*y=w174:dbl)
                n108 = Wait (ms)(milliseconds to wait=w174) -> ()  [unwired: 1 out]
                n109 = Unbundle By Name(w171) -> ("mortor設定"=w167:T5)
                n110 = Index Array(array=w167, index=3) -> (element=w170:T6)
                n111 = call "__move_motor2.vi"("Moving distance"=-50, "motor setup"=w170) -> ()  [unwired: 2 in, 2 out]
              }
              frame #8 {
                # "５：データーC/C"
                n112 = local read "1Dデータ"() -> (w177:dbl[])
                n113 = Unbundle By Name(w179) -> ("P.M.aveg"=w183:i32)
                n114 = Index Array(array=w177, index=0) -> (element=w181:dbl)
                n115 = call "__READ_PM_1ch_E4419A_aveg.VI"("aveg"=w183, "frq(GHz)"=w181, "GPIB"=w175) -> ("chA"=w180:dbl)  [unwired: 4 in]
                n116 = Replace Array Subset(array=w177, new element=w180, index=5) -> (w176:dbl[])
                n117 = local write "1Dデータ"(w176) -> ()
              }
              frame #9 {
                n118 = local read "1Dデータ"() -> (w184:dbl[])
              }
            }
          }
        }
      }
    }
  }
  n119 = stacked-sequence {
    tunnel: w6 -> [_ w190 w210]
    frame #0 {
      n120 = local read "Control"() -> (w187:T2)
      n121 = local read "SBRAクラスタ"() -> (w188:T4)
      n122 = Unbundle By Name(w187) -> ("Th"=w185:dbl, "Tc"=w189:dbl)
      n123 = Bundle By Name(cluster=w188, "Th"=w185, "Tc"=w189) -> (w186:T4)
      n124 = local write "SBRAクラスタ"(w186) -> ()
    }
    frame #1 {
      n125 = call "___2ddata_to_multigraph.vi"("列"=i32[] [0, 1, 2, 3, 4, 5], "データ配列"=w190) -> ("XYグラフ"=→"XYグラフ 4":cluster{"データ配列":dbl[], "データ配列":dbl[]}[])  [unwired: 5 in]
    }
    frame #2 {
      n126 = local read "SBR_Set"() -> (w211:T3)
      n127 = local read "Control"() -> (w206:T2)
      n128 = Unbundle By Name(w211) -> ("P/V         V/P"=w197:bool)
      n129 = Unbundle By Name(w206) -> ("DATAパス"=w205:path, "FreqLO"=w198:dbl, "Th"=w196:dbl, "Tc"=w195:dbl, "MPI offset(mm)"=w194:dbl)
      n130 = Unbundle By Name(w211) -> ("file_name"=w209:string)
      n131 = Transpose 2D Array(2D array=w210) -> (transposed array=w207:dbl[][])
      n132 = call "___save_2d_data_with_header.vi"("配列"=w207, "file_name"=w209, "パス"=w205) -> ("出力パス"=w208:path)  [unwired: 8 in]
      n133 = Strip Path(path=w208) -> (stripped path=w203:path, name=w202:string)
      n134 = local read "SBRAクラスタ"() -> (w204:T4)
      n135 = Bundle By Name(cluster=w204, "パス"=w203, "file_name"=w202, "LO(GHz)"=w198, "Offset(mm)"=w194, "P/V         V/P"=w197, "Th"=w196, "Tc"=w195) -> (w201:T4)
      n136 = call "__SBR_Ana2.vi"("SBRAクラスタ"=w201) -> ("XYグラフ 6"=→"XYグラフ 3":cluster{"データ配列":dbl[], "データ配列":dbl[]}[], "XYグラフ 9"=→"XYグラフ 5":cluster{"データ配列":dbl[], "データ配列":dbl[]}[], "XYグラフ 5"=→"XYグラフ 2":cluster{"データ配列":dbl[], "データ配列":dbl[]}[])  [unwired: 6 in]
    }
  }
